vi "__Is Path a Link.vi"(7 "Path in":path) -> (3 "Link?":bool, 8 "Path out":path, 14 "Exists?":bool)   [LabVIEW 2011]
doc: "This VI checks if the input path is a link (having an extension of .lnk) or a physical file, and if the path exists."
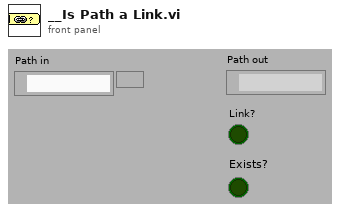
[diagram p1: front panel]
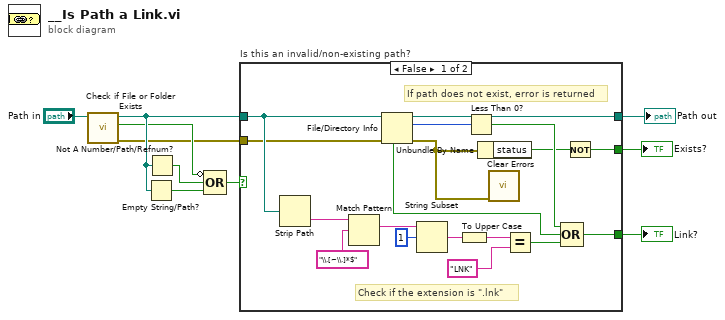
[diagram p0: block diagram]
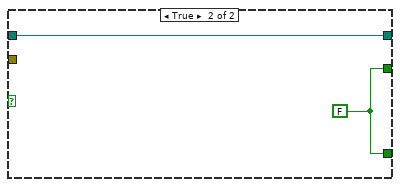
[diagram p2: hidden frame]
diagram:
  n1 = call <vilib>:"Check if File or Folder Exists.vi"("path"="Path in") -> ("error out"=w1:errorcluster, "file or folder exists?"=w2:bool, "dup path"=w3:path)  [unwired: 8 in]
  n2 = Empty String/Path?(string/path=w3) -> (empty?=w7:bool)
  n3 = Not A Number/Path/Refnum?(number/path/refnum=w3) -> (NaN/Path/Refnum?=w8:bool)
  n4 = Compound Arithmetic op=OR(invert w2, w8, w7) -> (w6:bool)
  n5 = case "Is this an invalid/non-existing path?" shown="False" w6 {
    tunnel: w3 -> [w21 w30]
    tunnel: [w20 w30] -> w10
    tunnel: [w17 w29] -> w9
    tunnel: [w11 w29] -> w5
    tunnel: w1 -> [w13 _]
    frame False {
      # "If path does not exist, error is returned"
      # "Check if the extension is \".lnk\""
      n6 = Strip Path(path=w21) -> (name=w27:string)  [unwired: 1 out]
      n7 = Match Pattern(string=w27, regular expression="\\.[~\\.]*$") -> (match substring=w25:string)  [unwired: 4 out]
      n8 = File/Directory Info(path=w21, error in=w13) -> (path out=w20:path, size=w16:i64, error out=w14:errorcluster, shortcut=w18:bool)  [unwired: 3 out]
      n9 = String Subset(string=w25, offset (0)=1) -> (substring=w24:string)  [unwired: 1 out]
      n10 = To Upper Case(1:w24) -> (0:w23:string)
      n11 = Less Than 0?(x=w16) -> (x < 0?=w15:bool)
      n12 = Unbundle By Name(w14) -> ("status"=w12:bool)
      n13 = call <vilib>:"Clear Errors.vi"("error in (no error)"=w14) -> ()  [unwired: 6 in, 1 out]
      n14 = Equal?(x=w23, y="LNK") -> (x = y?=w19:bool)
      n15 = Compound Arithmetic op=OR(w15, w18, w19) -> (w17:bool)
      n16 = Not(x=w12) -> (.not. x?=w11:bool)
    }
    frame True {
      w29 = FALSE
    }
  }
  "Path out" <- w10
  "Link?" <- w9
  "Exists?" <- w5
